vi "Laboratory PC Instrument.vi"() -> ()   [LabVIEW 2021]
panel:
  in  "Delay Time (s)":dbl=2.5
  in  "Delete .zip?":bool=TRUE
  in  "STOP":bool
  in  "Enable Output (T: Enable)":bool=TRUE
  in  "Output Channel (1: Channel 1)":i32(ring)=1 items=["Channel 1"=1, "Channel 2"=2]
  in  "VISA resource name":refnum<visa-resource-name>
  out "Handled queries":string[](array[string])
  out "UserData":string[](array[string])
  out "UserIDs":string[](array[string])
  out "Body":string
  out "error out":errorcluster
  in  "error in (no error)":errorcluster
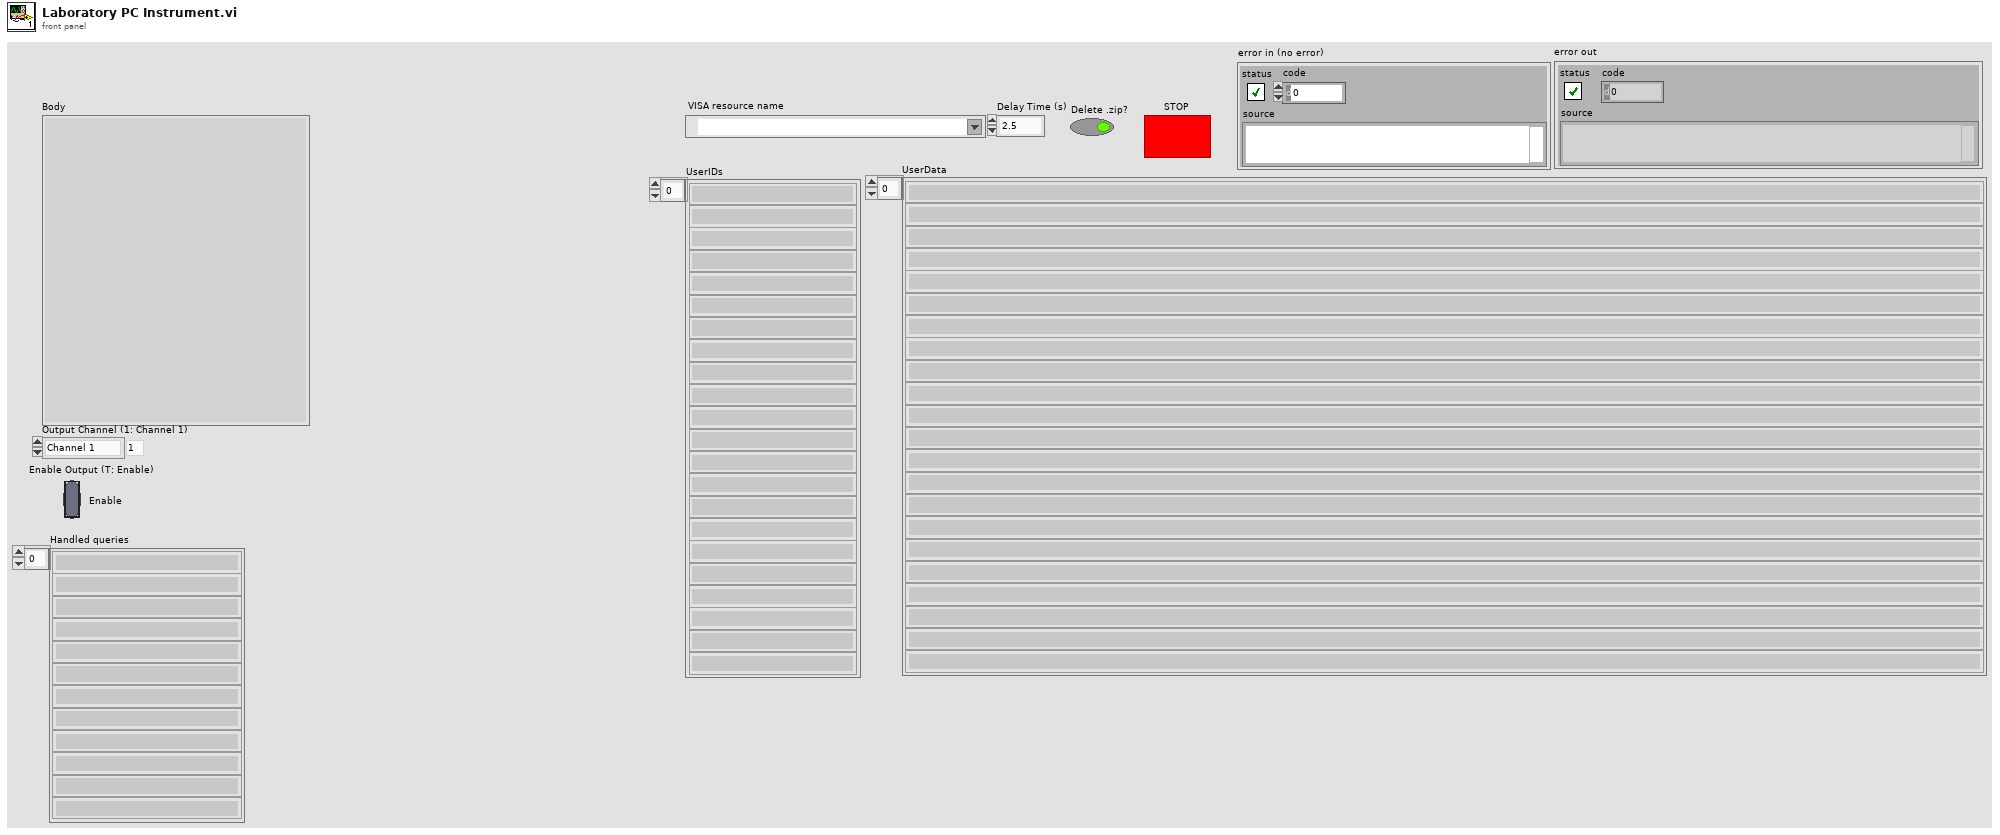
[diagram p1: front panel]
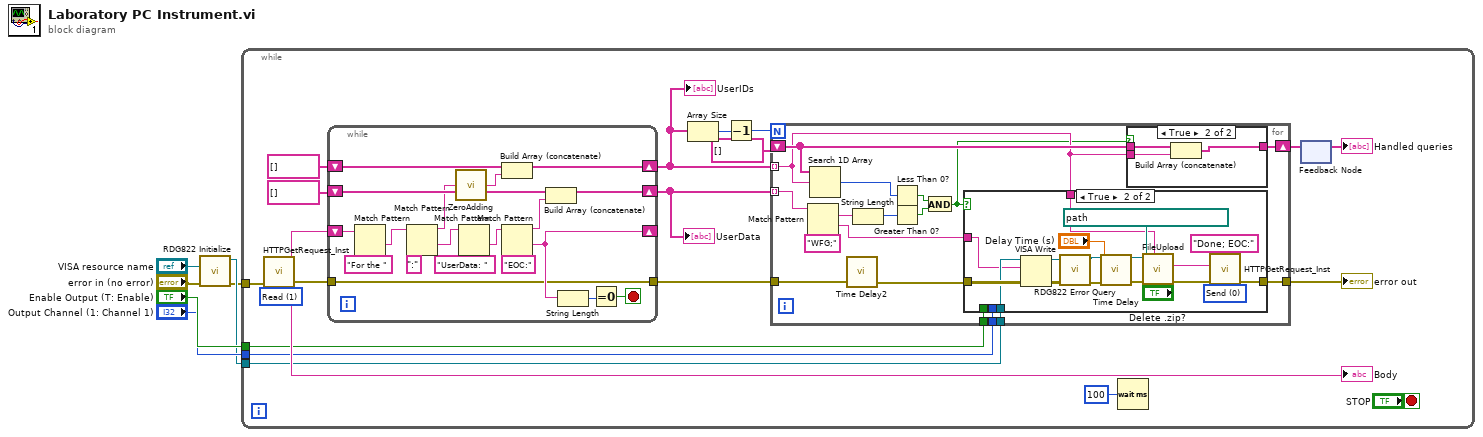
[diagram p0: block diagram]
diagram:
  n1 = call "RDG822 Initialize.vi"("error in (no error)"="error in (no error)", "VISA resource name"="VISA resource name") -> ("error out"=w1:errorcluster, "VISA resource name out"=w2:refnum<visa-resource-name>)  [unwired: 8 in]
  n2 = while {
    tunnel: "Enable Output (T: Enable)" -> [w16]
    tunnel: "Output Channel (1: Channel 1)" -> [w15]
    tunnel: w2 -> [w14]
    tunnel: w1 -> [w13]
    stop <- "STOP" stop-if-true
    w11 = u16 1 items=["Send", "Read", "Download", "Remove"] ("Send/Read/Download/Remove")
    n3 = call "HTTPGetRequest_Inst.vi"("Send/Read/Download/Remove"=w11, "error in (no error)"=w13) -> ("error out"=w23:errorcluster, "Body"=w26:string)  [unwired: 7 in, 1 out]
    "Body" <- w26
    n4 = while {
      shift-right: [w73] -> _
      shift-left: w26 -> [w68]
      shift-right: [w79] -> w8
      shift-left: string[] [] -> [w78]
      shift-right: [w71] -> w22
      shift-left: string[] [] -> [w70]
      tunnel: w23 -> [w69]
      tunnel: [w69] -> w21
      stop <- w83 stop-if-true
      n5 = Match Pattern(string=w68, regular expression="For the ") -> (after substring=w81:string)  [unwired: 1 in, 3 out]
      n6 = Match Pattern(string=w81, regular expression=":") -> (before substring=w67:string, after substring=w77:string)  [unwired: 1 in, 2 out]
      n7 = call "ZeroAdding.vi"("userID"=w67) -> ("zeroFilled_userID"=w66:string)
      n8 = Match Pattern(string=w77, regular expression="UserData: ") -> (after substring=w75:string)  [unwired: 1 in, 3 out]
      n9 = Build Array (concatenate)(w78, w66) -> (w79:string[])
      n10 = Match Pattern(string=w75, regular expression="EOC:") -> (before substring=w72:string, after substring=w73:string)  [unwired: 1 in, 2 out]
      n11 = Build Array (concatenate)(w70, w72) -> (w71:string[])
      n12 = String Length(string=w73) -> (length=w82:i32)
      n13 = Equal To 0?(x=w82) -> (x = 0?=w83:bool)
    }
    "UserIDs" <- w8
    "UserData" <- w22
    n14 = Array Size(array=w8) -> (size(s)=w19:i32)
    n15 = Decrement(x=w19) -> (x-1=w17:i32)
    n16 = for {
      N: w17 -> [_]
      tunnel: w8 -> [w35] mode=indexing
      tunnel: w22 -> [w30] mode=indexing
      tunnel: w21 -> [w43]
      tunnel: [w44] -> w20
      shift-right: [w41] -> w18
      shift-left: string[] [] -> [w39]
      tunnel: w16 -> [w38]
      tunnel: w15 -> [w37]
      tunnel: w14 -> [w36]
      n17 = Match Pattern(string=w30, regular expression="WFG;") -> (match substring=w27:string, after substring=w32:string)  [unwired: 1 in, 2 out]
      n18 = Search 1D Array(1D array=w39, element=w35) -> (index of element=w40:i32)  [unwired: 1 in]
      n19 = call "Time Delay2"("error in (no error)"=w43) -> ("error out"=w42:errorcluster)  [unwired: 10 in]
      n20 = String Length(string=w27) -> (length=w28:i32)
      n21 = Less Than 0?(x=w40) -> (x < 0?=w33:bool)
      n22 = Greater Than 0?(x=w28) -> (x > 0?=w29:bool)
      n23 = And(x=w33, y=w29) -> (x .and. y?=w34:bool)
      n24 = case shown="True" w34 {
        tunnel: w42 -> [w49 w65]
        tunnel: [w49 w53] -> w44
        tunnel: w32 -> [_ w55]
        tunnel: w38 -> [_ _]
        tunnel: w37 -> [_ _]
        tunnel: w36 -> [_ w64]
        tunnel: w35 -> [_ w52]
        frame False {
        }
        frame True {
          w54 = u16 0 items=["Send", "Read", "Download", "Remove"] ("Send/Read/Download/Remove")
          n25 = VISA Write(VISA resource name=w64, write buffer=w55, error in (no error)=w65) -> (VISA resource name out=w62:refnum<visa-resource-name>, error out=w63:errorcluster)  [unwired: 1 out]
          n26 = call "RDG822 Error Query.vi"("error in (no error)"=w63, "VISA resource name"=w62) -> ("error out"=w59:errorcluster, "VISA resource name out"=w60:refnum<visa-resource-name>)  [unwired: 6 in, 2 out]
          n27 = call "Time Delay"("error in (no error)"=w59, "Delay Time (s)"="Delay Time (s)") -> ("error out"=w61:errorcluster)  [unwired: 9 in]
          n28 = call "FileUpload.vi"("FileName"=w52, "error in"=w61, "Delete .zip?"="Delete .zip?", "Zip path"=path "E:/Study/НИР_Маг/Archives", "VISA resource name"=w60) -> ("error out"=w50:errorcluster)  [unwired: 6 in]
          n29 = call "HTTPGetRequest_Inst.vi"("Send/Read/Download/Remove"=w54, "error in (no error)"=w50, "userdata="="Done; EOC:", "ReqNum"=w52) -> ("error out"=w53:errorcluster)  [unwired: 5 in, 2 out]
        }
      }
      n30 = case shown="True" w34 {
        tunnel: w39 -> [w45 w48]
        tunnel: [w45 w47] -> w41
        tunnel: w35 -> [_ w46]
        frame False {
        }
        frame True {
          n31 = Build Array (concatenate)(w48, w46) -> (w47:string[])
        }
      }
    }
    "error out" <- w20
    n32 = Wait (ms)(milliseconds to wait=u32 100) -> ()  [unwired: 1 out]
    n33 = feedback #1() -> (→"Handled queries":string[])  [unwired: 1 in]
    n34 = feedback-in #1(w18) -> ()
  }
